vi "Add_Trailing_Slash.vi"(1 "Wanted? (True)":bool=TRUE, 2 "path":string) -> (0 "path with trailing slash":string)   [LabVIEW 2019, in "ByteREST.lvlib" / "RESTBase.lvclass"]
uses:
  RESTBase.lvclass
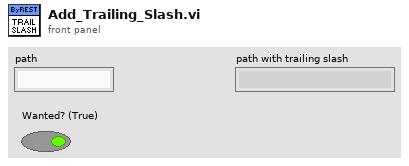
[diagram p1: front panel]
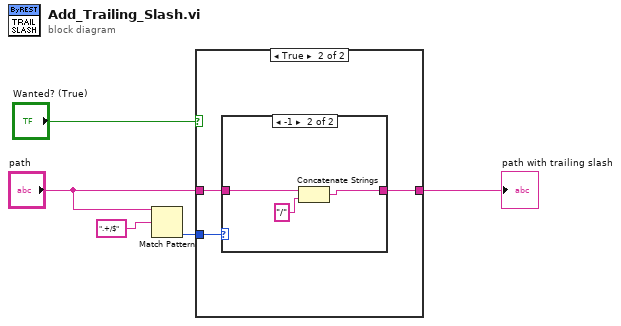
[diagram p0: block diagram]
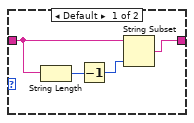
[diagram p3: hidden frame]
diagram:
  n1 = Match Pattern(string="path", regular expression=".+/$") -> (offset past match=w5:i32)  [unwired: 1 in, 3 out]
  n2 = case shown="True" "Wanted? (True)" {
    tunnel: w5 -> [w8 w16]
    tunnel: "path" -> [w6 w15]
    tunnel: [w7 w14] -> w2
    frame False {
      n3 = case shown="-1" w8 {
        tunnel: [w10 w13] -> w7
        tunnel: w6 -> [w12 w13]
        frame Default {
          n4 = String Length(string=w12) -> (length=w9:i32)
          n5 = Decrement(x=w9) -> (x-1=w11:i32)
          n6 = String Subset(string=w12, length (rest)=w11) -> (substring=w10:string)  [unwired: 1 in]
        }
        frame -1 {
        }
      }
    }
    frame True {
      n7 = case shown="-1" w16 {
        tunnel: w15 -> [w17 w20]
        tunnel: [w17 w18] -> w14
        frame Default {
        }
        frame -1 {
          n8 = Concatenate Strings(w20, "/" ("string")) -> (w18:string)
        }
      }
    }
  }
  "path with trailing slash" <- w2
